vi "Highlight execution example.vi"() -> ()   [LabVIEW 2010]
panel:
  in  "Number 6":dbl=6.0
  in  "Number 5":dbl=5.0
  in  "Number 4":dbl=4.0
  in  "Number 3":dbl=3.0
  out "Result":dbl=231.0
  in  "Number 2":dbl=2.0
  in  "Number 1":dbl=1.0
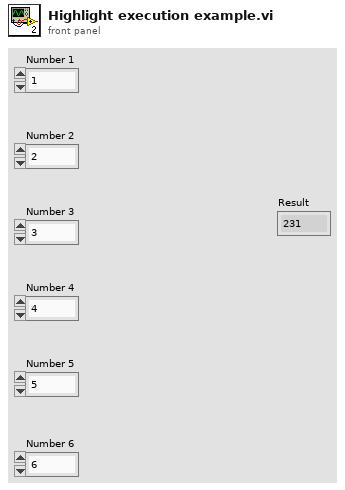
[diagram p1: front panel]
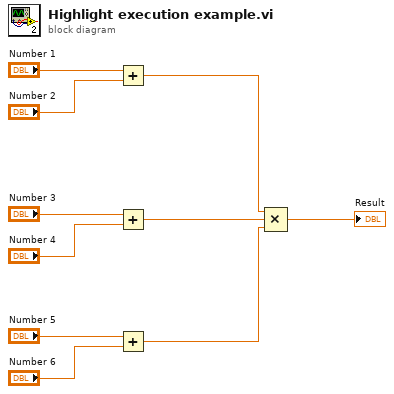
[diagram p0: block diagram]
diagram:
  n1 = Add(x="Number 1", y="Number 2") -> (x+y=w4:dbl)
  n2 = Add(x="Number 3", y="Number 4") -> (x+y=w3:dbl)
  n3 = Add(x="Number 5", y="Number 6") -> (x+y=w2:dbl)
  n4 = Compound Arithmetic op=MULTIPLY(w4, w3, w2) -> (→"Result":dbl)
